vi "testare.vi"() -> ()   [LabVIEW 2024]
uses:
  <vilib>/National Instruments/NI Super Simple Neural Networks/Neural Network.lvclass
panel:
  out "new picture":picture
  out "Rezultat":string
  in  "pen 2":T1={"Width"=10, "Style"=enum."Solid"}
  in  "stop":bool
  in  "Refresh Button":bool
  out "Clasificare clase":cluster{string, "Numeric Control":dbl}[](array[cluster])
  out "image 28x28":sgl[][](graph)
  out "picture":picture
  out "pen":T1={"Width"=1, "Style"=enum."Solid"}
  in  "NN-Configuratie":path
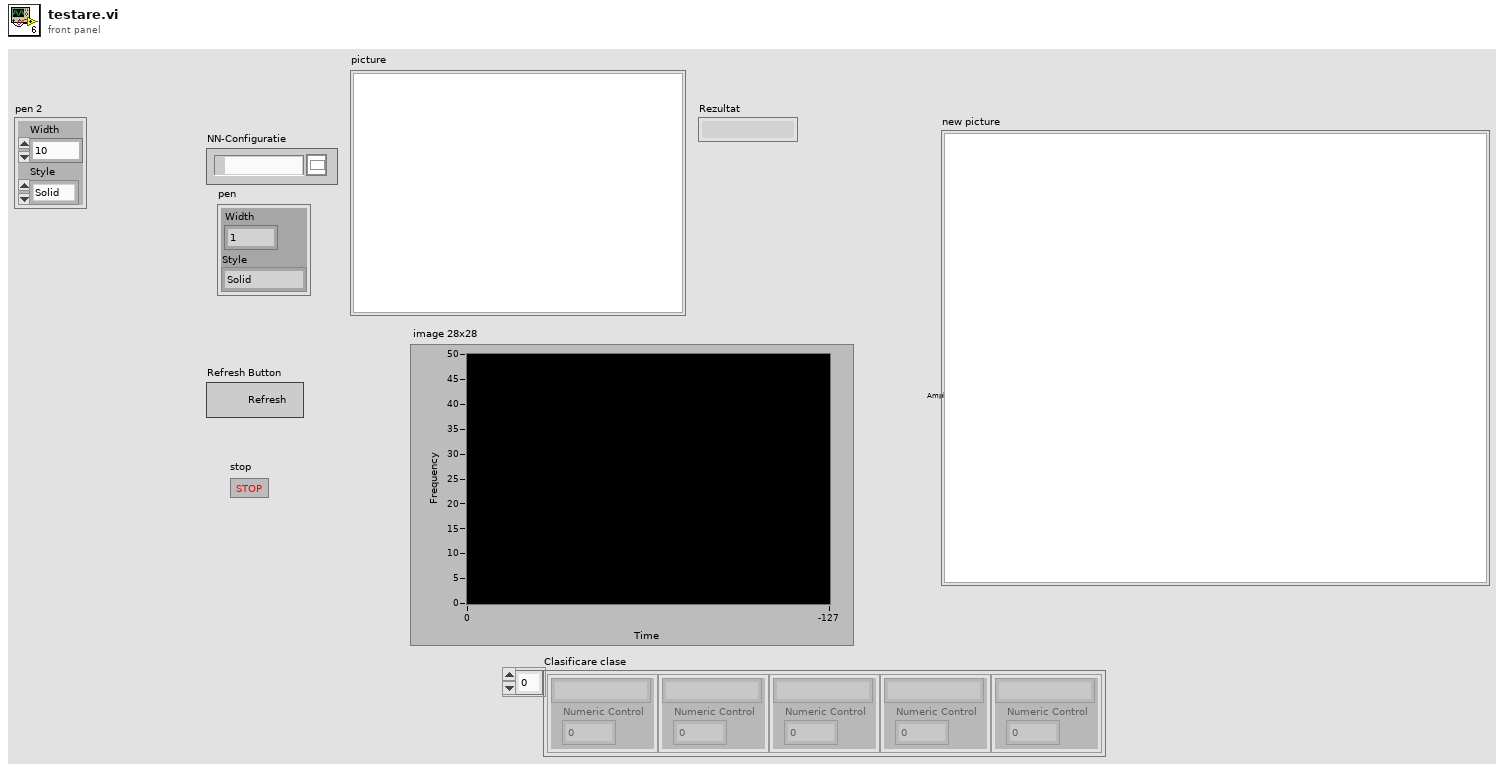
[diagram p1: front panel]
types:
  T1 = cluster{"Width":u16, "Style":enum32{"Solid", "Dash", "Dot", "DashDot", "DashDotDot"}}
  T2 = cluster{"left":i16, "top":i16, "right":i16, "bottom":i16}
  T3 = typedef "LVMouseTypeDef.ctl" = cluster{"Mouse Position":cluster{"X":i32, "Y":i32}, "Mouse Modifiers":cluster{"Button Down":bool, "Shift Mod":bool, "Menu Mod":bool, "Option Mod":bool}}
  T4 = typedef "imagedata.ctl" = cluster{"image type":i32, "image depth":i32, "image":u8[], "mask":u8[], "colors":u32[], "Rectangle":cluster{"left":i16, "top":i16, "right":i16, "bottom":i16}}
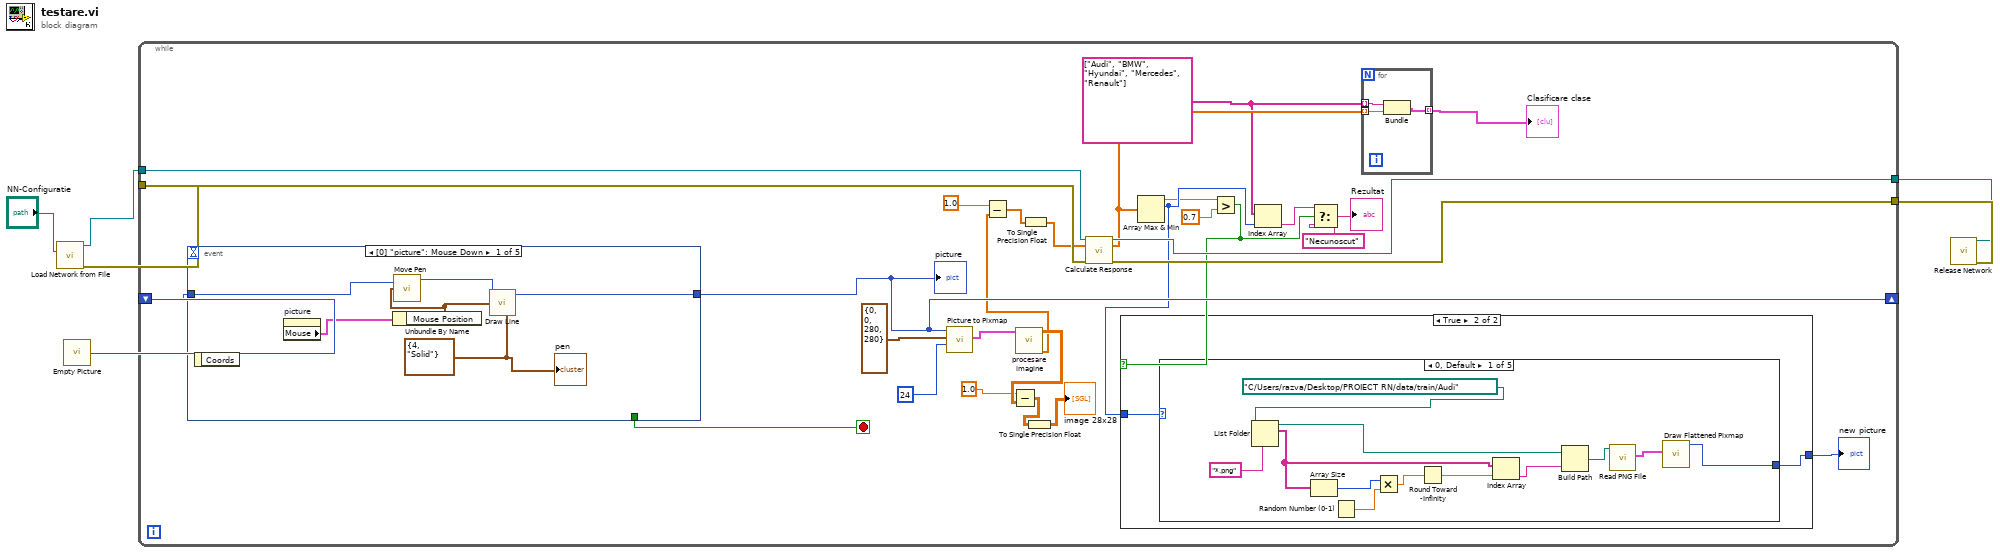
[diagram p0: block diagram]
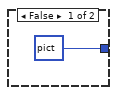
[diagram p2: hidden frame]
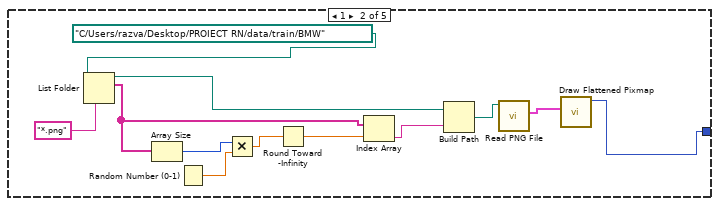
[diagram p3: hidden frame]
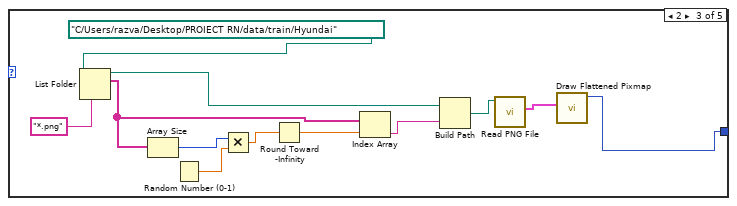
[diagram p4: hidden frame]
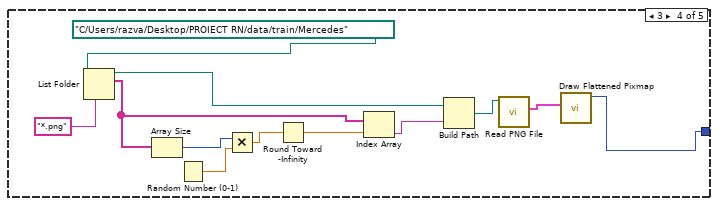
[diagram p5: hidden frame]
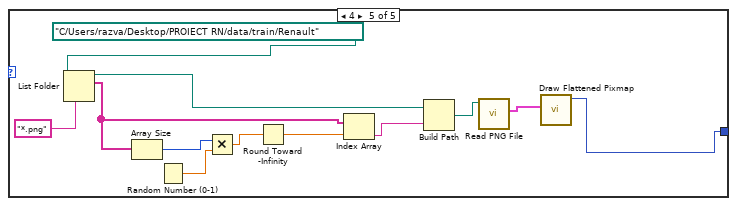
[diagram p6: hidden frame]
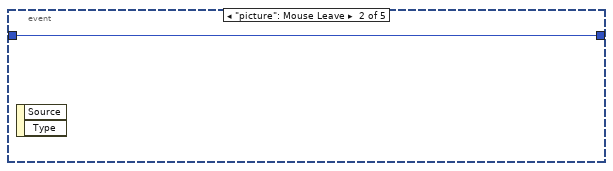
[diagram p7: hidden frame]
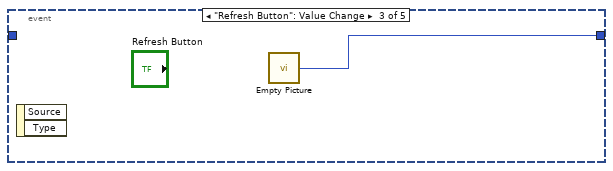
[diagram p8: hidden frame]
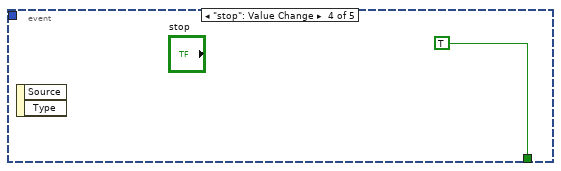
[diagram p9: hidden frame]
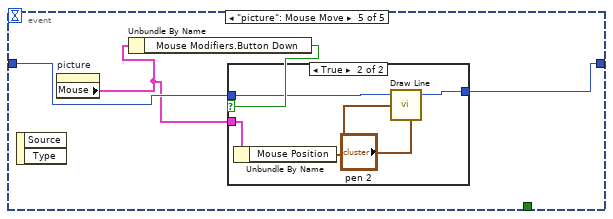
[diagram p10: hidden frame]
diagram:
  n1 = call <vilib>:"Load Network from File.vi"("File Path (dialog)"="NN-Configuratie") -> ("Neural Network Out"=w3:refnum<class "Neural Network.lvclass">, "Error Out"=w4:errorcluster)  [unwired: 11 in, 2 out]
  n2 = call "Empty Picture"() -> ("empty picture"=w5:picture)
  n3 = while {
    shift-right: [w25] -> _
    shift-left: w5 -> [w35]
    tunnel: w4 -> [w31]
    tunnel: w3 -> [w30]
    tunnel: [w27] -> w2
    tunnel: [w26] -> w1
    stop <- w29 stop-if-true
    w19 = string[] ["Audi", "BMW", "Hyundai", "Mercedes", "Renault"]
    n4 = event shown="[0] \"picture\": Mouse Down" {
      selector: _ -> [_ _ _ _ _]
      dyn-events: _ -> [_ _ _ _ _]
      timeout: _ -> [_ _ _ _ _]
      tunnel: w35 -> [w107 w108 _ _ w113]
      tunnel: [w105 w108 w109 _ w112] -> w25
      tunnel: [_ _ _ TRUE _] -> w29
      event "picture": Mouse Down {
        w104 = T1 {"Width"=4, "Style"=enum."Solid"} ("pen")
        n5 = event-data() -> ()  [unwired: 1 in, 1 out]
        n6 = property on="picture" class="Pict"() -> ("Mouse"=w103:T3)  [unwired: 2 in, 2 out]
        n7 = Unbundle By Name(w103) -> ("Mouse Position"=w102:cluster{"X":i32, "Y":i32})
        n8 = call <vilib>:"Move Pen.vi"("new position"=w102, "picture"=w107) -> ("new picture"=w106:picture)  [unwired: 3 in]
        n9 = call <vilib>:"Draw Line.vi"("picture"=w106, "end point"=w102, "pen"=w104) -> ("new picture"=w105:picture)  [unwired: 6 in]
        "pen" <- w104
      }
      event "picture": Mouse Leave {
        n10 = event-data() -> ()  [unwired: 1 in, 2 out]
      }
      event "Refresh Button": Value Change {
        n11 = event-data() -> ()  [unwired: 1 in, 2 out]
        n12 = call "Empty Picture"() -> ("empty picture"=w109:picture)
      }
      event "stop": Value Change {
        n13 = event-data() -> ()  [unwired: 1 in, 2 out]
      }
      event "picture": Mouse Move {
        n14 = event-data() -> ()  [unwired: 1 in, 2 out]
        n15 = property on="picture" class="Pict"() -> ("Mouse"=w111:T3)  [unwired: 2 in, 2 out]
        n16 = Unbundle By Name(w111) -> ("Mouse Modifiers.Button Down"=w114:bool)
        n17 = case shown="True" w114 {
          tunnel: w113 -> [w115 w118]
          tunnel: w111 -> [_ w116]
          tunnel: [w115 w117] -> w112
          frame False {
          }
          frame True {
            n18 = Unbundle By Name(w116) -> ("Mouse Position"=w119:cluster{"X":i32, "Y":i32})
            n19 = call <vilib>:"Draw Line.vi"("picture"=w118, "end point"=w119, "pen"="pen 2") -> ("new picture"=w117:picture)  [unwired: 6 in]
          }
        }
      }
    }
    "picture" <- w25
    n20 = call <vilib>:"Picture to Pixmap.vi"("depth"=24, "rect"=T2 {"left"=0, "top"=0, "right"=280, "bottom"=280}, "picture"=w25) -> ("image data"=w32:T4)  [unwired: 7 in, 1 out]
    n21 = call "procesare imagine.vi"("image data"=w32) -> ("image array"=w10:sgl[], "image 28x28"=w16:sgl[][])  [unwired: 9 in]
    n22 = Subtract(x=1.0, y=w10) -> (x-y=w8:dbl[])
    n23 = Subtract(x=1.0, y=w16) -> (x-y=w14:dbl[][])
    n24 = To Single Precision Float(number=w8) -> (single precision float=w7:sgl[])
    n25 = To Single Precision Float(number=w14) -> (single precision float=→"image 28x28":sgl[][])
    n26 = call <vilib>:"Calculate Response.vi"("Neural Network In"=w30, "Inputs"=w7, "Error In"=w31) -> ("Neural Network Out"=w26:refnum<class "Neural Network.lvclass">, "Outputs"=w24:dbl[], "Error Out"=w27:errorcluster)  [unwired: 10 in]
    n27 = Array Max & Min(array=w24) -> (max value=w11:dbl, max index (indices)=w12:i32)  [unwired: 2 out]
    n28 = Greater?(x=w11, y=0.7) -> (0:w17:bool)
    n29 = case shown="True" w17 {
      tunnel: [picture data[5B] ("new picture") w38] -> w18
      tunnel: w12 -> [_ w37]
      frame False {
      }
      frame True {
        n30 = case shown="0, Default" w37 {
          tunnel: [w40 w52 w64 w76 w88] -> w38
          frame 0, Default {
            n31 = List Folder(path=path "C:/Users/razva/Desktop/PROIECT RN/data/train/Audi", pattern="*.png") -> (path out=w44:path, filenames=w39:string[])  [unwired: 2 in, 2 out]
            n32 = Array Size(array=w39) -> (size(s)=w48:i32)
            n33 = Random Number (0-1)() -> (number: 0 to 1=w47:dbl)
            n34 = Multiply(x=w48, y=w47) -> (x*y=w46:dbl)
            n35 = Round Toward -Infinity(1:w46) -> (0:w45:dbl)
            n36 = Index Array(array=w39, index=w45) -> (element=w43:string)
            n37 = Build Path(base path=w44, name or relative path=w43) -> (appended path=w42:path)
            n38 = call <vilib>:"Read PNG File.vi"("path to PNG file"=w42) -> ("image data"=w41:T4)  [unwired: 8 in, 2 out]
            n39 = call <vilib>:"Draw Flattened Pixmap.vi"("image data"=w41) -> ("new picture"=w40:picture)  [unwired: 8 in]
          }
          frame 1 {
            n40 = List Folder(path=path "C:/Users/razva/Desktop/PROIECT RN/data/train/BMW", pattern="*.png") -> (path out=w56:path, filenames=w51:string[])  [unwired: 2 in, 2 out]
            n41 = Array Size(array=w51) -> (size(s)=w60:i32)
            n42 = Random Number (0-1)() -> (number: 0 to 1=w59:dbl)
            n43 = Multiply(x=w60, y=w59) -> (x*y=w58:dbl)
            n44 = Round Toward -Infinity(1:w58) -> (0:w57:dbl)
            n45 = Index Array(array=w51, index=w57) -> (element=w55:string)
            n46 = Build Path(base path=w56, name or relative path=w55) -> (appended path=w54:path)
            n47 = call <vilib>:"Read PNG File.vi"("path to PNG file"=w54) -> ("image data"=w53:T4)  [unwired: 8 in, 2 out]
            n48 = call <vilib>:"Draw Flattened Pixmap.vi"("image data"=w53) -> ("new picture"=w52:picture)  [unwired: 8 in]
          }
          frame 2 {
            n49 = List Folder(path=path "C:/Users/razva/Desktop/PROIECT RN/data/train/Hyundai", pattern="*.png") -> (path out=w68:path, filenames=w63:string[])  [unwired: 2 in, 2 out]
            n50 = Array Size(array=w63) -> (size(s)=w72:i32)
            n51 = Random Number (0-1)() -> (number: 0 to 1=w71:dbl)
            n52 = Multiply(x=w72, y=w71) -> (x*y=w70:dbl)
            n53 = Round Toward -Infinity(1:w70) -> (0:w69:dbl)
            n54 = Index Array(array=w63, index=w69) -> (element=w67:string)
            n55 = Build Path(base path=w68, name or relative path=w67) -> (appended path=w66:path)
            n56 = call <vilib>:"Read PNG File.vi"("path to PNG file"=w66) -> ("image data"=w65:T4)  [unwired: 8 in, 2 out]
            n57 = call <vilib>:"Draw Flattened Pixmap.vi"("image data"=w65) -> ("new picture"=w64:picture)  [unwired: 8 in]
          }
          frame 3 {
            n58 = List Folder(path=path "C:/Users/razva/Desktop/PROIECT RN/data/train/Mercedes", pattern="*.png") -> (path out=w80:path, filenames=w75:string[])  [unwired: 2 in, 2 out]
            n59 = Array Size(array=w75) -> (size(s)=w84:i32)
            n60 = Random Number (0-1)() -> (number: 0 to 1=w83:dbl)
            n61 = Multiply(x=w84, y=w83) -> (x*y=w82:dbl)
            n62 = Round Toward -Infinity(1:w82) -> (0:w81:dbl)
            n63 = Index Array(array=w75, index=w81) -> (element=w79:string)
            n64 = Build Path(base path=w80, name or relative path=w79) -> (appended path=w78:path)
            n65 = call <vilib>:"Read PNG File.vi"("path to PNG file"=w78) -> ("image data"=w77:T4)  [unwired: 8 in, 2 out]
            n66 = call <vilib>:"Draw Flattened Pixmap.vi"("image data"=w77) -> ("new picture"=w76:picture)  [unwired: 8 in]
          }
          frame 4 {
            n67 = List Folder(path=path "C:/Users/razva/Desktop/PROIECT RN/data/train/Renault", pattern="*.png") -> (path out=w92:path, filenames=w87:string[])  [unwired: 2 in, 2 out]
            n68 = Array Size(array=w87) -> (size(s)=w96:i32)
            n69 = Random Number (0-1)() -> (number: 0 to 1=w95:dbl)
            n70 = Multiply(x=w96, y=w95) -> (x*y=w94:dbl)
            n71 = Round Toward -Infinity(1:w94) -> (0:w93:dbl)
            n72 = Index Array(array=w87, index=w93) -> (element=w91:string)
            n73 = Build Path(base path=w92, name or relative path=w91) -> (appended path=w90:path)
            n74 = call <vilib>:"Read PNG File.vi"("path to PNG file"=w90) -> ("image data"=w89:T4)  [unwired: 8 in, 2 out]
            n75 = call <vilib>:"Draw Flattened Pixmap.vi"("image data"=w89) -> ("new picture"=w88:picture)  [unwired: 8 in]
          }
        }
      }
    }
    "new picture" <- w18
    n76 = Index Array(array=w19, index=w12) -> (element=w22:string)
    n77 = Select(t=w22, s=w17, f="Necunoscut") -> (s? t:f=→"Rezultat":string)
    n78 = for {
      tunnel: w24 -> [w101] mode=indexing
      tunnel: w19 -> [w100] mode=indexing
      tunnel: [w99] -> w28 mode=indexing
      n79 = Bundle(w100, "Numeric Control"=w101) -> (w99:cluster{string, "Numeric Control":dbl})  [unwired: 1 in]
    }
    "Clasificare clase" <- w28
  }
  n80 = call <vilib>:"Release Network.vi"("Neural Network"=w1, "Error In"=w2) -> ()  [unwired: 13 in, 1 out]
